vi "set_multiramp_soak_profile_segment_soak_process_value.vi"(8 "error in (no error)":errorcluster, 9 "Soak value (C)":dbl, 10 "Segment number":u8 max=15, 11 "connection ID":refnum<k5>) -> (0 "error out":errorcluster, 3 "connection ID out":refnum<k5>)   [LabVIEW 2018]
panel:
  out "bytes written":i32
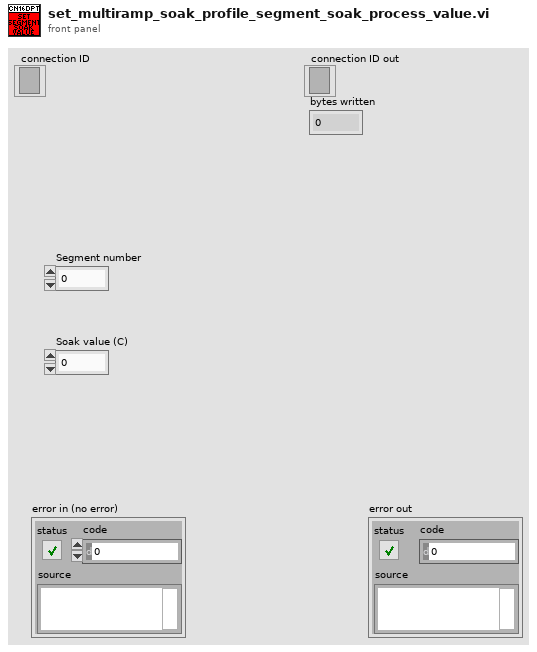
[diagram p1: front panel]
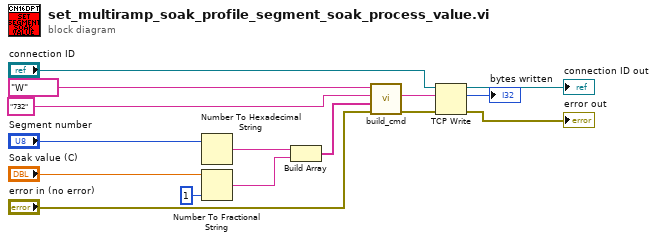
[diagram p0: block diagram]
diagram:
  n1 = Number To Hexadecimal String(2:"Segment number") -> (0:w7:string)  [unwired: 1 in]
  n2 = Number To Fractional String(number="Soak value (C)", precision (6)=i16 1) -> (F-format string=w6:string)  [unwired: 2 in]
  n3 = Build Array(w7, w6) -> (w9:string[])
  n4 = call "build_cmd.vi"("error in (no error)"="error in (no error)", "Parameter list"=w9, "Command ID"="732", "Command class"="W") -> ("error out"=w12:errorcluster, "Command"=w11:string)  [unwired: 6 in]
  n5 = TCP Write(connection ID="connection ID", data in=w11, error in (no error)=w12) -> (connection ID out=→"connection ID out":refnum<k5>, bytes written=→"bytes written":i32, error out=→"error out":errorcluster)  [unwired: 1 in]
